vi "Get Map Values Array.vi"(0 "DBMap in":refnum<class "DBMap.lvclass">, 11 "error in (no error)":errorcluster {"code" format="Error %.0f"}) -> (4 "DBMap out":refnum<class "DBMap.lvclass">, 6 "Map Array":T1(array[numeric]), 15 "error out":errorcluster {"code" format="Error %.0f"})   [LabVIEW 2024, in "DBMap.lvclass"]
uses:
  DBMap.lvclass
  DBMap.lvclass/DBMap.ctl
  <vilib>/drjdpowell/SQLite Library/SQLite.lvlib
  <vilib>/drjdpowell/SQLite Library/SQL Connection/Execute SQL (1D String).vi
  <vilib>/drjdpowell/SQLite Library/SQL Connection/Connection.lvclass
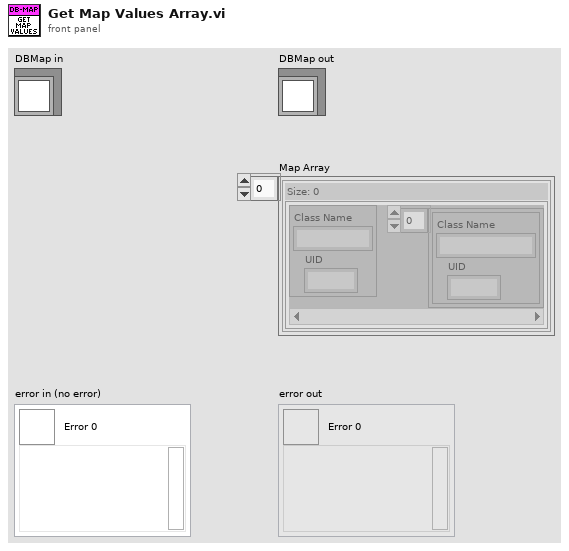
[diagram p1: front panel]
types:
  T1 = map{cluster{"Class Name":string, "UID":i32}, cluster{"Class Name":string, "UID":i32}[]}[]
  T2 = map{cluster{"Class Name":string, "UID":i32}, cluster{"Class Name":string, "UID":i32}[]}
  T3 = typedef "Semaphore RefNum" = refnum<k1>
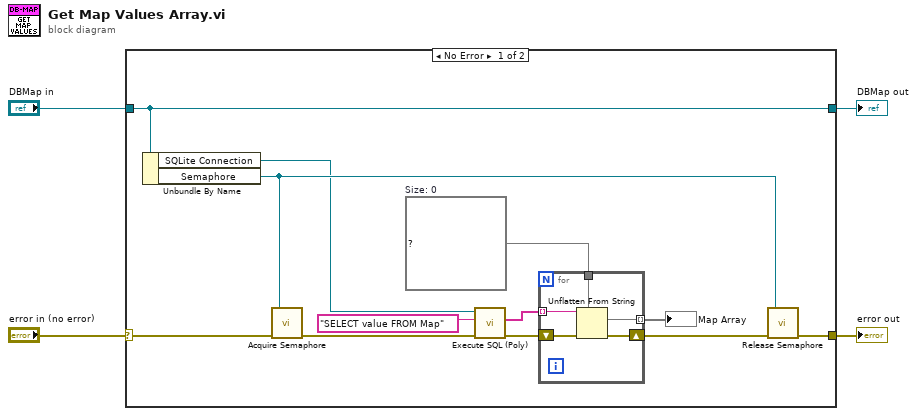
[diagram p0: block diagram]
diagram:
  n1 = case shown="No Error" "error in (no error)" {
    selector: "error in (no error)" -> [w15 w23]
    tunnel: [w14 w23] -> w3
    tunnel: [w16 w22] -> w1
    tunnel: "DBMap in" -> [w16 w22]
    frame No Error {
      w10 = T2 {}  # Size: 0
      n2 = Unbundle By Name(w16) -> ("SQLite Connection"=w5:refnum<class "Connection.lvclass">, "Semaphore"=w13:T3)
      n3 = call <vilib>:"Acquire Semaphore.vi"("error in (no error)"=w15, "semaphore"=w13) -> ("error out"=w7:errorcluster)  [unwired: 3 in, 2 out]
      n4 = call-poly <vilib>:"Execute SQL (Poly).vi"("error in (no error)"=w7, "SQL"="SELECT value FROM Map", "SQLite Connection in"=w5) -> ("error out"=w11:errorcluster, "Result Set"=w9:string[])  [unwired: 5 in, 2 out]
      n5 = for {
        shift-right: [w20] -> w6
        shift-left: w11 -> [w21]
        tunnel: w10 -> [w18]
        tunnel: w9 -> [w19] mode=indexing
        tunnel: [w17] -> w8 mode=indexing
        n6 = Unflatten From String(type=w18, binary string=w19, error in (no error)=w21) -> (value=w17:T2, error out=w20:errorcluster)  [unwired: 2 in, 1 out]
      }
      "Map Array" <- w8
      n7 = call <vilib>:"Release Semaphore.vi"("error in (no error)"=w6, "semaphore"=w13) -> ("error out"=w14:errorcluster)  [unwired: 4 in, 1 out]
    }
    frame Error {
    }
  }
  "error out" <- w3
  "DBMap out" <- w1
